vi "Get Accuracy.vi"(11 "Stand in":refnum<class "Stand.lvclass">) -> (2 "Accuracy [MPa]":dbl)   [LabVIEW 2019, in "Stand.lvclass"]
uses:
  Stand.lvclass
  Stand.lvclass/Stand.ctl
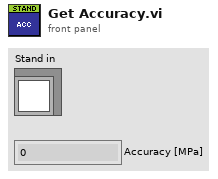
[diagram p1: front panel]
types:
  T1 = typedef "Direction.ctl" = enum8{"DUT", "Chamber"}
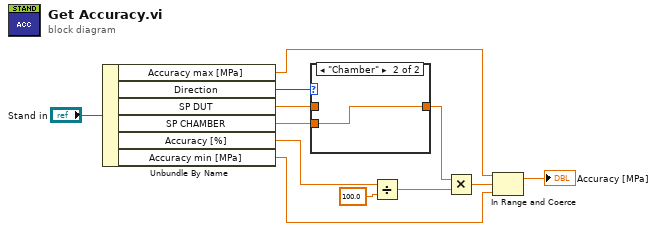
[diagram p0: block diagram]
diagram:
  n1 = Unbundle By Name("Stand in") -> ("Accuracy max [MPa]"=w1:dbl, "Direction"=w11:T1, "SP DUT"=w9:dbl, "SP CHAMBER"=w10:dbl, "Accuracy [%]"=w8:dbl, "Accuracy min [MPa]"=w3:dbl)
  n2 = case shown="\"Chamber\"" w11 {
    tunnel: [w13 w14] -> w6
    tunnel: w10 -> [_ w14]
    tunnel: w9 -> [w13 _]
    frame "DUT" {
    }
    frame "Chamber" {
    }
  }
  n3 = Divide(x=w8, y=100.0) -> (x/y=w5:dbl)
  n4 = Multiply(x=w6, y=w5) -> (x*y=w4:dbl)
  n5 = In Range and Coerce(upper limit=w1, x=w4, lower limit=w3) -> (coerced(x)=→"Accuracy [MPa]":dbl)  [unwired: 1 out]
